vi "Korektur Hystereseschleife.vi"(8 "error in (no error)":errorcluster, 9 "Input Array":dbl[](array[numeric])) -> (0 "error out":errorcluster, 1 "Output Array":dbl[](array[numeric]))   [LabVIEW 2016]
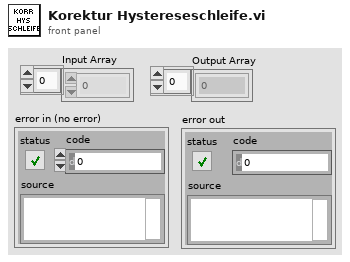
[diagram p1: front panel]
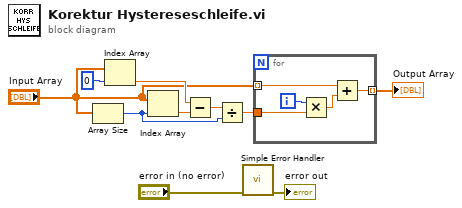
[diagram p0: block diagram]
diagram:
  n1 = Array Size(array="Input Array") -> (size(s)=w4:i32)
  n2 = Index Array(array="Input Array", index=0) -> (element=w8:dbl)
  n3 = Index Array(array="Input Array", index=w4) -> (element=w7:dbl)
  n4 = Subtract(x=w8, y=w7) -> (x-y=w5:dbl)
  n5 = Divide(x=w5, y=w4) -> (x/y=w3:dbl)
  n6 = call <vilib>:"Simple Error Handler.vi"("error in (no error)"="error in (no error)") -> ("error out"=→"error out":errorcluster)  [unwired: 4 in, 4 out]
  n7 = for {
    tunnel: "Input Array" -> [w12] mode=indexing
    tunnel: [w11] -> w10 mode=indexing
    tunnel: w3 -> [w13]
    i -> [w14]
    n8 = Multiply(x=w14, y=w13) -> (x*y=w15:dbl)
    n9 = Add(x=w12, y=w15) -> (x+y=w11:dbl)
  }
  "Output Array" <- w10
